vi "Get X and Y (multiple).vi"(8 "error in (no error)":errorcluster, 11 "XY-data":cluster{"X-array":dbl[], "Y-array":dbl[]}[](array[cluster]) {"Y-array" format="%.2p"; "X-array" format="%.2p"}) -> (0 "error out":errorcluster, 1 "Y-Arrays":cluster{"Y-array":dbl[]}[](array[cluster]), 2 "X-Arrays":cluster{"X-array":dbl[]}[](array[cluster]), 3 "XY-data out":cluster{"X-array":dbl[], "Y-array":dbl[]}[](array[cluster]) {"Y-array" format="%.2p"; "X-array" format="%.2p"})   [LabVIEW 2016, in "xy_utilities.lvlib"]
doc: "Returns the X and Y arrays contained in <b>XY-data</b>.\n\nWire data to the data input to determine the polymorphic instance to use or manually select the instance."
uses:
  xy_utilities.lvlib
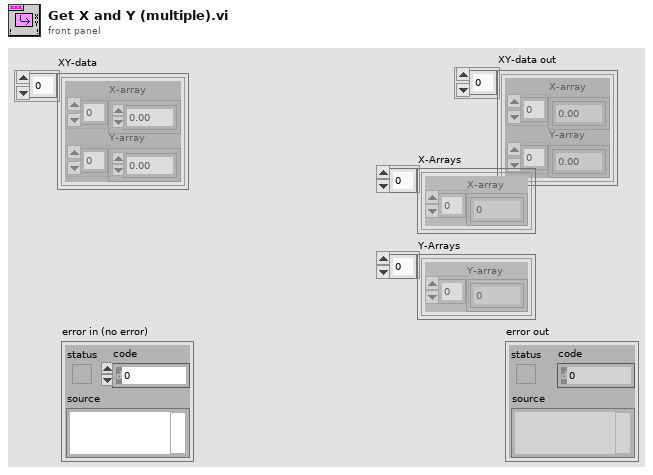
[diagram p1: front panel]
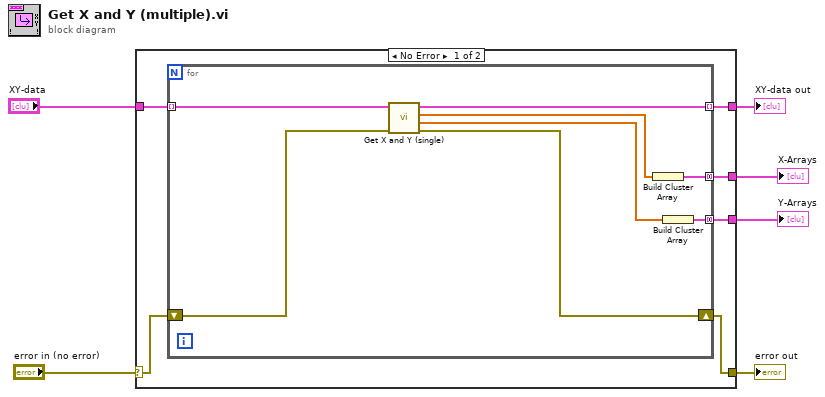
[diagram p0: block diagram]
diagram:
  n1 = case shown="No Error" "error in (no error)" {
    selector: "error in (no error)" -> [w10 w22]
    tunnel: [w9 w22] -> w5
    tunnel: "XY-data" -> [w12 w21]
    tunnel: [w11 w21] -> w3
    tunnel: [w8 _] -> w2
    tunnel: [w7 _] -> w1
    frame No Error {
      n2 = for {
        tunnel: w12 -> [w20] mode=indexing
        tunnel: [w19] -> w11 mode=indexing
        shift-right: [w17] -> w9
        shift-left: w10 -> [w18]
        tunnel: [w13] -> w8 mode=concatenating
        tunnel: [w14] -> w7 mode=concatenating
        n3 = call "Get X and Y (single).vi"("error in (no error)"=w18, "XY-data"=w20) -> ("error out"=w17:errorcluster, "Y-array"=w15:dbl[], "X-array"=w16:dbl[], "XY-data out"=w19:cluster{"X-array":dbl[], "Y-array":dbl[]})  [unwired: 6 in]
        n4 = Build Cluster Array(w16) -> (w13:cluster{"X-array":dbl[]}[])
        n5 = Build Cluster Array(w15) -> (w14:cluster{"Y-array":dbl[]}[])
      }
    }
    frame Error {
    }
  }
  "error out" <- w5
  "XY-data out" <- w3
  "X-Arrays" <- w2
  "Y-Arrays" <- w1
